vi "Is File Changed.vi"(8 "path":path, 10 "Default on First Call":bool) -> (3 "Changed":bool)   [LabVIEW 2014]
panel:
  in  "last mod":timestamp
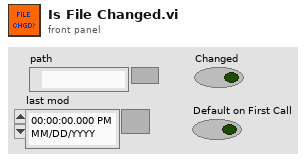
[diagram p1: front panel]
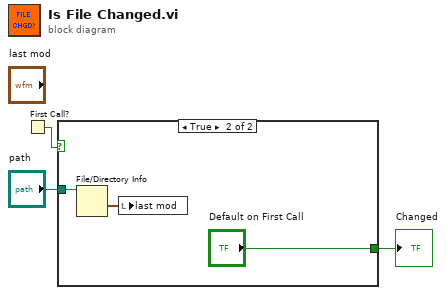
[diagram p0: block diagram]
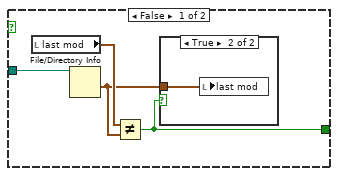
[diagram p2: hidden frame]
diagram:
  n1 = First Call?() -> (First Call?: T/F=w3:bool)
  n2 = case shown="True" w3 {
    tunnel: [w5 "Default on First Call"] -> w1
    tunnel: "path" -> [w7 w9]
    frame False {
      n3 = local read "last mod"() -> (w6:timestamp)
      n4 = File/Directory Info(path=w7) -> (last mod=w4:timestamp)  [unwired: 1 in, 6 out]
      n5 = Not Equal?(x=w6, y=w4) -> (x != y?=w5:bool)
      n6 = case shown="True" w5 {
        tunnel: w4 -> [_ w8]
        frame False {
        }
        frame True {
          n7 = local write "last mod"(w8) -> ()
        }
      }
    }
    frame True {
      n8 = File/Directory Info(path=w9) -> (last mod=w10:timestamp)  [unwired: 1 in, 6 out]
      n9 = local write "last mod"(w10) -> ()
    }
  }
  "Changed" <- w1
